vi "Write AVG Filter type.vi"(8 "error in (no error)":errorcluster, 10 "AVG Filter type":T1, 11 "ElectrometerInternalConfiguration in":refnum<class "ElectrometerInternalConfiguration.lvclass">) -> (0 "error out":errorcluster, 3 "ElectrometerInternalConfiguration out":refnum<class "ElectrometerInternalConfiguration.lvclass">)   [LabVIEW 2016, in "ElectrometerInternalConfiguration.lvclass"]
uses:
  ElectrometerInternalConfiguration.lvclass
  Electrometer/AVG Filter type.ctl
  ElectrometerInternalConfiguration.lvclass/ElectrometerInternalConfiguration.ctl
  Electrometer/Electrometer.lvclass
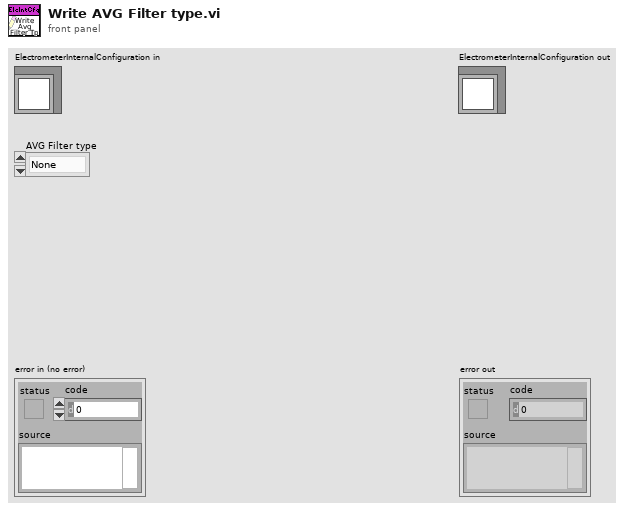
[diagram p1: front panel]
types:
  T1 = typedef "Electrometer.lvclass/AVG Filter type.ctl" = enum16{"None", "Scalar", "Advanced"}
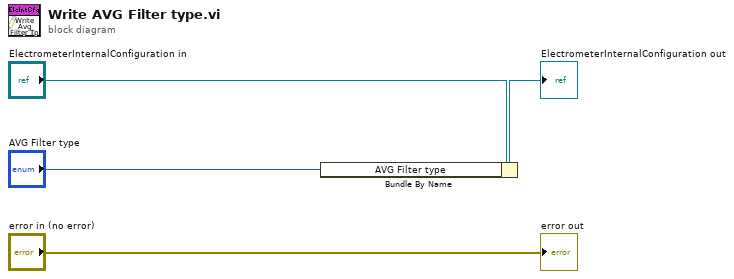
[diagram p0: block diagram]
diagram:
  n1 = Bundle By Name(cluster="ElectrometerInternalConfiguration in", "AVG Filter type"="AVG Filter type") -> (→"ElectrometerInternalConfiguration out":refnum<class "ElectrometerInternalConfiguration.lvclass">)
  "error out" <- "error in (no error)"
